vi "Set Temperature.vi"(8 "error in (no error)":errorcluster, 11 "CCDCamera in":refnum<class "Real Camera.lvclass">) -> (0 "error out":errorcluster, 3 "CCDCamera out":refnum<class "Real Camera.lvclass">)   [LabVIEW 2018, in "Real Camera.lvclass"]
doc: "Set the CCD temperature"
uses:
  Real Camera.lvclass
  C:/Users/Denis/Desktop/S4ACS/S4ACS/Simulated_CCD_Camera/Simulated Camera.lvclass
  Simulated_CCD_Camera/Simulated Camera.lvclass
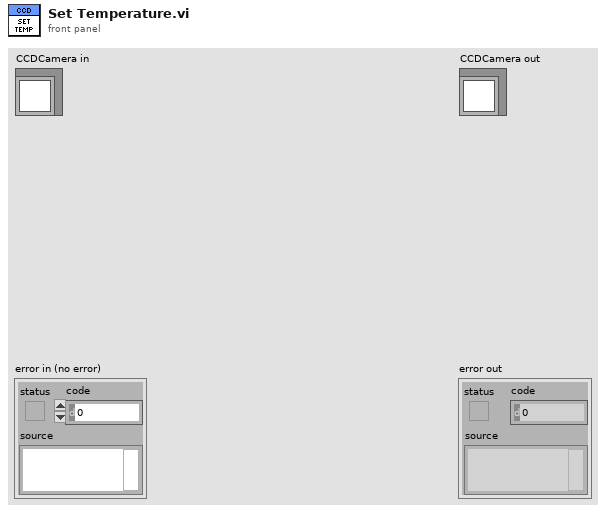
[diagram p1: front panel]
types:
  T1 = cluster{"COOLER_POWER_STATUS":u16, "TEMP":i32, "EXPTIME":dbl, "#FRAMES":u32, "#CYCLES":u32, "#SEQS":u32, "WAVEPLATE_POS":u16}
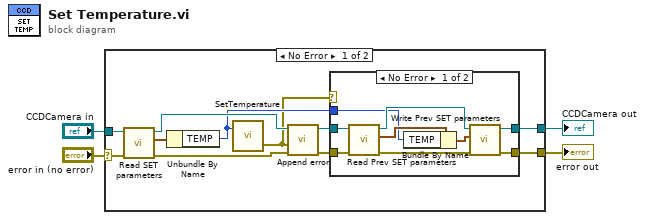
[diagram p0: block diagram]
diagram:
  n1 = case shown="No Error" "error in (no error)" {
    selector: "error in (no error)" -> [w15 w27]
    tunnel: "CCDCamera in" -> [w13 w28]
    tunnel: [w8 w28] -> w1
    tunnel: [w7 w27] -> w4
    frame No Error {
      n2 = call-dynamic "Read SET parameters.vi"("error in (no error)"=w15, "Simulated_CCD_Camera in"=w13) -> ("error out"=w11:errorcluster, "New SET parameters"=w14:T1, "Simulated_CCD_Camera out"=w12:refnum<class "Real Camera.lvclass">)  [unwired: 7 in]
      n3 = Unbundle By Name(w14) -> ("TEMP"=w6:i32)
      n4 = call <userlib>:"SetTemperature.vi"("temperature"=w6) -> ("error out"=w5:errorcluster)  [unwired: 1 in, 1 out]
      n5 = call "Append error.vi"("error in (no error)"=w11, "error"=w5, "Simulated_CCD_Camera in"=w12) -> ("error out"=w9:errorcluster, "Simulated_CCD_Camera out"=w10:refnum<class "Real Camera.lvclass">)  [unwired: 7 in]
      n6 = case shown="No Error" w5 {
        tunnel: [w24 w26] -> w8
        tunnel: [w23 w25] -> w7
        tunnel: w10 -> [w19 w26]
        tunnel: w9 -> [w20 w25]
        tunnel: w6 -> [w16 _]
        frame No Error {
          n7 = call-dynamic "Read Prev SET parameters.vi"("error in (no error)"=w20, "Simulated_CCD_Camera in"=w19) -> ("error out"=w21:errorcluster, "Prev SET parameters"=w18:T1, "Simulated_CCD_Camera out"=w22:refnum<class "Real Camera.lvclass">)  [unwired: 7 in]
          n8 = Bundle By Name(cluster=w18, "TEMP"=w16) -> (w17:T1)
          n9 = call-dynamic "Write Prev SET parameters.vi"("error in (no error)"=w21, "Prev SET parameters"=w17, "Simulated_CCD_Camera in"=w22) -> ("error out"=w23:errorcluster, "Simulated_CCD_Camera out"=w24:refnum<class "Real Camera.lvclass">)  [unwired: 7 in]
        }
        frame Error {
        }
      }
    }
    frame Error {
    }
  }
  "error out" <- w4
  "CCDCamera out" <- w1
